vi "Examine Waveform Data Type.vi"() -> ()   [LabVIEW 2019]
panel:
  out "Waveform Graph":waveform(dbl)(graph)
  in  "Waveform":waveform(dbl)={"t0"=timestamp(3638070250 s since 1904-01-01), "dt"=0.1, "Y"=[0.0, 0.587785, 0.951057, 0.951057, 0.587785, 0.0, -0.587785, -0.951057, -0.951057, -0.587785, 0.0]}
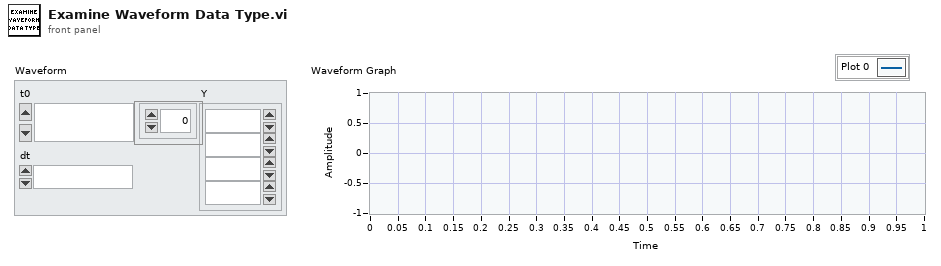
[diagram p1: front panel]
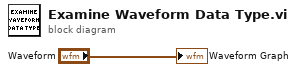
[diagram p0: block diagram]
diagram:
  "Waveform Graph" <- "Waveform"
